vi "Constant - Default UDP Port Number.vi"() -> (3 "port":u16=30303)   [LabVIEW 2021]
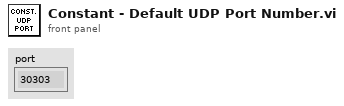
[diagram p1: front panel]
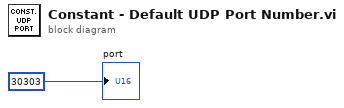
[diagram p0: block diagram]
diagram:
  "port" <- u16 30303 ("port")
